vi "Allocate IO.vi"(8 "error in (no error)":errorcluster) -> (0 "error out":errorcluster, 2 "IO":T1, 3 "Blackboard out":refnum<class "Blackboard.lvclass">)   [LabVIEW 2021, in "Car Wash Support.lvlib"]
uses:
  Car Wash Support.lvlib
  IO Refs.ctl
  <vilib>/TSA/Abstract Data Classes/Abs_Types/Boolean/Abs_Boolean.lvclass
  <vilib>/TSA/Abstract Data Classes/Abs_Types/I32 Integer/Abs_I32 Integer.lvclass
  <vilib>/TSA/Abstract Data Classes/Abs_Types/Double Float/Abs_Double Float.lvclass
  <vilib>/TSA/Event Log/Event_TextLog/Event_TextLog.lvclass
  C:/Program Files (x86)/National Instruments/LabVIEW 2021/vi.lib/TSA/Event Log/abs_EventLog/abs_EventLog.lvclass
  Wash Indicators.ctl
  Wash Options.ctl
  Blackboard/Blackboard.lvclass
  <vilib>/TSA/Event Log/abs_EventLog/Support/Severity Code.ctl
  <vilib>/TSA/Event Log/abs_EventLog/abs_EventLog.lvclass/abs_EventLog.ctl
  Blackboard/Blackboard.lvclass/Blackboard.ctl
  Blackboard/Get Value Type/Get Boolean.vi
  Blackboard/Get Value Type/Get I32.vi
  Blackboard/Get Value Type/Get DBL.vi
  <vilib>/TSA/Event Log/abs_EventLog/Properties/Write Severity Code.vi
  Blackboard/Support/Index Group.vi
  Blackboard/Support/Index Tags.vi
  <vilib>/TSA/Omni-Bus/Local Bus/Support/Bool/Local Bus_Boolean.lvclass
  C:/Program Files (x86)/National Instruments/LabVIEW 2021/vi.lib/TSA/Abstract Data Classes/Abs_Types/Value/Abs_Value.lvclass
  <vilib>/TSA/Omni-Bus/Local Bus/Support/I32/Local Bus_I32.lvclass
  <vilib>/TSA/Omni-Bus/Local Bus/Support/DBL/Local Bus_DBL.lvclass
  <vilib>/TSA/Omni-Bus/Local Bus/Support/Initialise DVR's.vi
  <vilib>/TSA/Abstract Data Classes/Abs_Types/Value/Abs_Value.lvclass
  <vilib>/TSA/Abstract Data Classes/Abs_Types/Type/Abs_Type.lvclass
  <vilib>/TSA/Omni-Bus/Local Bus/Support/SGL/Local Bus_SGL.lvclass
  <vilib>/TSA/Omni-Bus/Local Bus/Support/EXT/Local Bus_EXT.lvclass
  <vilib>/TSA/Omni-Bus/Local Bus/Support/STR/Local Bus_String.lvclass
  <vilib>/TSA/Omni-Bus/Local Bus/Support/Variant/Local Bus_Variant.lvclass
  <vilib>/TSA/Omni-Bus/Local Bus/Support/WFM/Local Bus_Waveform.lvclass
  <vilib>/TSA/Omni-Bus/Local Bus/Support/Time/Local Bus_Time.lvclass
  <vilib>/TSA/Omni-Bus/Local Bus/Support/U8/Local Bus_U8.lvclass
  <vilib>/TSA/Omni-Bus/Local Bus/Support/U16/Local Bus_U16.lvclass
  <vilib>/TSA/Omni-Bus/Local Bus/Support/U32/Local Bus_U32.lvclass
  <vilib>/TSA/Omni-Bus/Local Bus/Support/U64/Local Bus_U64.lvclass
  <vilib>/TSA/Omni-Bus/Local Bus/Support/I8/Local Bus_I8.lvclass
  <vilib>/TSA/Omni-Bus/Local Bus/Support/I16/Local Bus_I16.lvclass
  <vilib>/TSA/Omni-Bus/Local Bus/Support/I64/Local Bus_I64.lvclass
  <vilib>/TSA/Omni-Bus/Local Bus/Support/CSGL/Local Bus_CSGL.lvclass
  <vilib>/TSA/Omni-Bus/Local Bus/Support/CDBL/Local Bus_CDBL.lvclass
  <vilib>/TSA/Omni-Bus/Local Bus/Support/CEXT/Local Bus_CEXT.lvclass
  <vilib>/TSA/Omni-Bus/Local Bus/Support/Type/Local Bus_Type.lvclass
  <vilib>/TSA/Event Log/abs_EventLog/abs_EventLog.lvclass
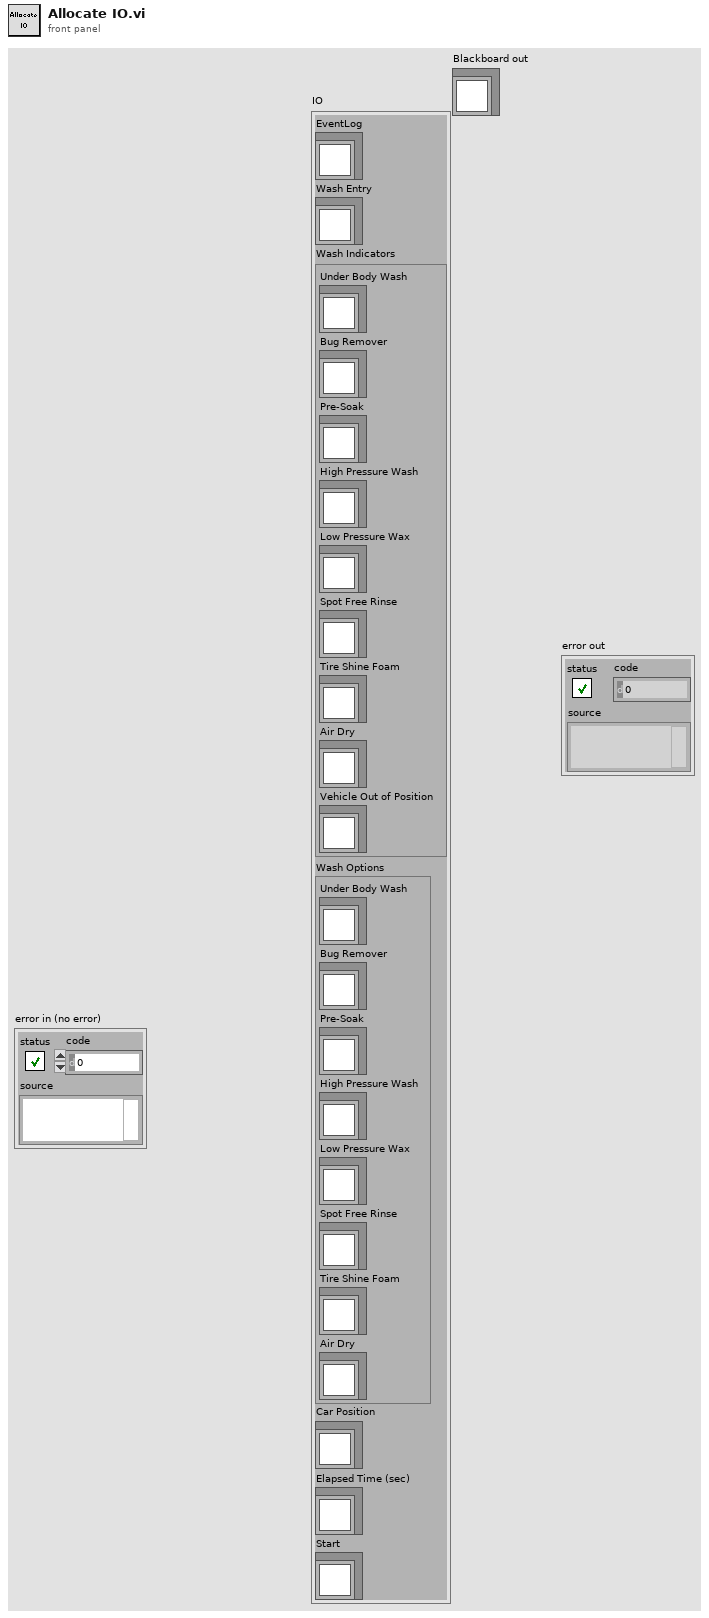
[diagram p1: front panel]
types:
  T1 = typedef "Car Wash Support.lvlib/IO Refs.ctl" = cluster{"EventLog":refnum<class "Event_TextLog.lvclass">, "Wash Entry":refnum<class "Abs_Boolean.lvclass">, "Wash Indicators":T2, "Wash Options":T3, "Car Position":refnum<class "Abs_I32 Integer.lvclass">, "Elapsed Time (sec)":refnum<class "Abs_Double Float.lvclass">, "Start":refnum<class "Abs_Boolean.lvclass">}
  T2 = typedef "Car Wash Support.lvlib/Wash Indicators.ctl" = cluster{"Under Body Wash":refnum<class "Abs_Boolean.lvclass">, "Bug Remover":refnum<class "Abs_Boolean.lvclass">, "Pre-Soak":refnum<class "Abs_Boolean.lvclass">, "High Pressure Wash":refnum<class "Abs_Boolean.lvclass">, "Low Pressure Wax":refnum<class "Abs_Boolean.lvclass">, "Spot Free Rinse":refnum<class "Abs_Boolean.lvclass">, "Tire Shine Foam":refnum<class "Abs_Boolean.lvclass">, "Air Dry":refnum<class "Abs_Boolean.lvclass">, "Vehicle Out of Position":refnum<class "Abs_Boolean.lvclass">}
  T3 = typedef "Car Wash Support.lvlib/Wash Options.ctl" = cluster{"Under Body Wash":refnum<class "Abs_Boolean.lvclass">, "Bug Remover":refnum<class "Abs_Boolean.lvclass">, "Pre-Soak":refnum<class "Abs_Boolean.lvclass">, "High Pressure Wash":refnum<class "Abs_Boolean.lvclass">, "Low Pressure Wax":refnum<class "Abs_Boolean.lvclass">, "Spot Free Rinse":refnum<class "Abs_Boolean.lvclass">, "Tire Shine Foam":refnum<class "Abs_Boolean.lvclass">, "Air Dry":refnum<class "Abs_Boolean.lvclass">}
  T4 = typedef "abs_EventLog.lvclass/Severity Code.ctl" = enum16{"emergency", "alert", "critical", "error", "warning", "notice", "info", "debug"}
  T5 = cluster{"[0]":refnum<class "Abs_Boolean.lvclass">, "[1]":refnum<class "Abs_Boolean.lvclass">, "[2]":refnum<class "Abs_Boolean.lvclass">, "[3]":refnum<class "Abs_Boolean.lvclass">, "[4]":refnum<class "Abs_Boolean.lvclass">, "[5]":refnum<class "Abs_Boolean.lvclass">, "[6]":refnum<class "Abs_Boolean.lvclass">, "[7]":refnum<class "Abs_Boolean.lvclass">, "[8]":refnum<class "Abs_Boolean.lvclass">}
  T6 = cluster{"[0]":refnum<class "Abs_Boolean.lvclass">, "[1]":refnum<class "Abs_Boolean.lvclass">, "[2]":refnum<class "Abs_Boolean.lvclass">, "[3]":refnum<class "Abs_Boolean.lvclass">, "[4]":refnum<class "Abs_Boolean.lvclass">, "[5]":refnum<class "Abs_Boolean.lvclass">, "[6]":refnum<class "Abs_Boolean.lvclass">, "[7]":refnum<class "Abs_Boolean.lvclass">}
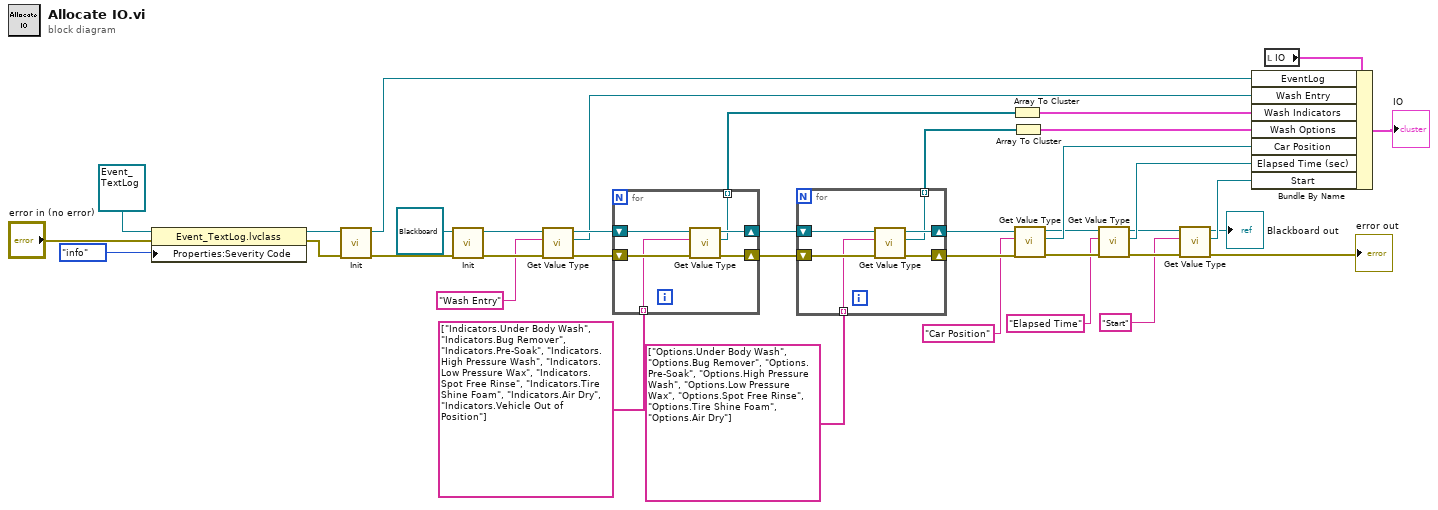
[diagram p0: block diagram]
diagram:
  n1 = property class="Event_TextLog.lvclass"(reference=refnum<class "Event_TextLog.lvclass"> refnum ("Event_TextLog in"), error in="error in (no error)", "Properties:Severity Code"=Severity_Code."info" ("Severity Code")) -> (reference out=w8:refnum<class "Event_TextLog.lvclass">, error out=w5:errorcluster)
  n2 = call-dynamic "Init.vi"("error in (no error)"=w5, "Event_TextLog in"=w8) -> ("error out"=w6:errorcluster, "Event_TextLog out"=w4:refnum<class "Event_TextLog.lvclass">)  [unwired: 8 in]
  n3 = call-dynamic "Init.vi"("error in (no error)"=w6, "bt_Blackboard in"=refnum<class "Blackboard.lvclass"> refnum) -> ("error out"=w37:errorcluster, "bt_Blackboard out"=w35:refnum<class "Blackboard.lvclass">)  [unwired: 8 in]
  n4 = call-poly "Get Value Type.vi"("error in (no error)"=w37, "Tag"="Wash Entry", "Blackboard in"=w35) -> ("error out"=w38:errorcluster, "Value"=w29:refnum<class "Abs_Boolean.lvclass">, "Blackboard out"=w36:refnum<class "Blackboard.lvclass">)  [unwired: 5 in, 1 out]
  n5 = for {
    tunnel: [w40] -> w28 mode=indexing
    shift-right: [w41] -> w33
    shift-left: w38 -> [w44]
    shift-right: [w42] -> w34
    shift-left: w36 -> [w43]
    tunnel: string[] ["Indicators.Under Body Wash", "Indicators.Bug Remover", "Indicators.Pre-Soak", "Indicators.High Pressure Wash", "Indicators.Low Pressure Wax", "Indicators.Spot Free Rinse", "Indicators.Tire Shine Foam", "Indicators.Air Dry", "Indicators.Vehicle Out of Position"] ("Array") -> [w39] mode=indexing
    n6 = call-poly "Get Value Type.vi"("error in (no error)"=w44, "Tag"=w39, "Blackboard in"=w43) -> ("error out"=w41:errorcluster, "Value"=w40:refnum<class "Abs_Boolean.lvclass">, "Blackboard out"=w42:refnum<class "Blackboard.lvclass">)  [unwired: 5 in, 1 out]
  }
  n7 = for {
    tunnel: [w46] -> w27 mode=indexing
    shift-right: [w48] -> w32
    shift-left: w34 -> [w50]
    shift-right: [w47] -> w31
    shift-left: w33 -> [w49]
    tunnel: string[] ["Options.Under Body Wash", "Options.Bug Remover", "Options.Pre-Soak", "Options.High Pressure Wash", "Options.Low Pressure Wax", "Options.Spot Free Rinse", "Options.Tire Shine Foam", "Options.Air Dry"] ("Array") -> [w45] mode=indexing
    n8 = call-poly "Get Value Type.vi"("error in (no error)"=w49, "Tag"=w45, "Blackboard in"=w50) -> ("error out"=w47:errorcluster, "Value"=w46:refnum<class "Abs_Boolean.lvclass">, "Blackboard out"=w48:refnum<class "Blackboard.lvclass">)  [unwired: 5 in, 1 out]
  }
  n9 = Array To Cluster(array=w28) -> (cluster=w23:T5)
  n10 = Array To Cluster(array=w27) -> (cluster=w24:T6)
  n11 = call-poly "Get Value Type.vi"("error in (no error)"=w31, "Tag"="Car Position", "Blackboard in"=w32) -> ("error out"=w16:errorcluster, "Value"=w26:refnum<class "Abs_I32 Integer.lvclass">, "Blackboard out"=w18:refnum<class "Blackboard.lvclass">)  [unwired: 5 in, 1 out]
  n12 = call-poly "Get Value Type.vi"("error in (no error)"=w16, "Tag"="Elapsed Time", "Blackboard in"=w18) -> ("error out"=w13:errorcluster, "Value"=w17:refnum<class "Abs_Double Float.lvclass">, "Blackboard out"=w14:refnum<class "Blackboard.lvclass">)  [unwired: 5 in, 1 out]
  n13 = call-poly "Get Value Type.vi"("error in (no error)"=w13, "Tag"="Start", "Blackboard in"=w14) -> ("error out"=→"error out":errorcluster, "Value"=w11:refnum<class "Abs_Boolean.lvclass">, "Blackboard out"=→"Blackboard out":refnum<class "Blackboard.lvclass">)  [unwired: 5 in, 1 out]
  n14 = local read "IO"() -> (w30:T1)
  n15 = Bundle By Name(cluster=w30, "EventLog"=w4, "Wash Entry"=w29, "Wash Indicators"=w23, "Wash Options"=w24, "Car Position"=w26, "Elapsed Time (sec)"=w17, "Start"=w11) -> (→"IO":T1)
